vi "RT.vi"() -> ()   [LabVIEW 2025]
uses:
  Cluster.ctl
  Enum.ctl
  Conn_state.ctl
  <vilib>/FPGAPlugInAG/myRIO-1900/niLvFpga_Open_myRIO-1900.vi
  <vilib>/rvi/interface/common/dynamic/niFpgaDynamicAddResources.vi
  <vilib>/Utility/error.llb/Error Cluster From Error Code.vi
  <vilib>/rvi/errors/niLvFpgaAdjustHostInterfaceError.vi
  <vilib>/FPGAPlugInAG/Dynamic/niLvFpga_Close_Dynamic.vi
  <vilib>/rvi/interface/nirviOpenFPGA/nirviOpenFPGA.xnode
  FPGA Bitfiles/andrzejkozdrowsk_FPGATarget_fpgamain_Nau7SJ+XEAg.lvbitx
  <vilib>/rvi/interface/nirviReadWriteControl/nirviReadWriteControl.xnode
  <vilib>/rvi/interface/nirviCloseFPGA/nirviCloseFPGA.xnode
  <vilib>/rvi/interface/Simulation/niFpgaSimulationCallBeginRW.vi
  <resource>/objmgr/ni.dex.rc
  NiFpgaLv.dll
panel:
  in  "Acc_delay":u16=500
  out "Is Connected":bool
  out "Stop":bool
  out "Acc_Data":i16[](graph)
  out "error out":errorcluster
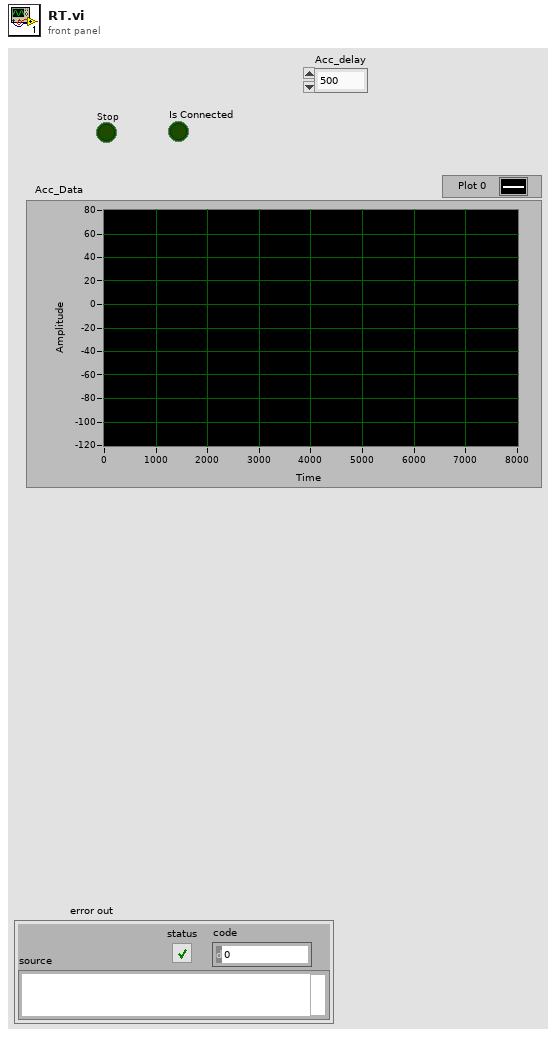
[diagram p1: front panel]
types:
  T1 = typedef "Conn_state.ctl" = enum16{"Disconected", "Reconecting", "Connected"}
  T2 = typedef "Cluster.ctl" = cluster{"X":u32, "Stop":bool, "Y":u32, "Z":u32, "Trigger":bool, "Select":T3}
  T3 = typedef "Enum.ctl" = enum16{"Trigger", "Stop", "Z", "Y", "X"}
  T4 = cluster{"Threshold_X":i16, "Threshold_Y":i16, "Threshold_Z":i16, "Trigger":bool}
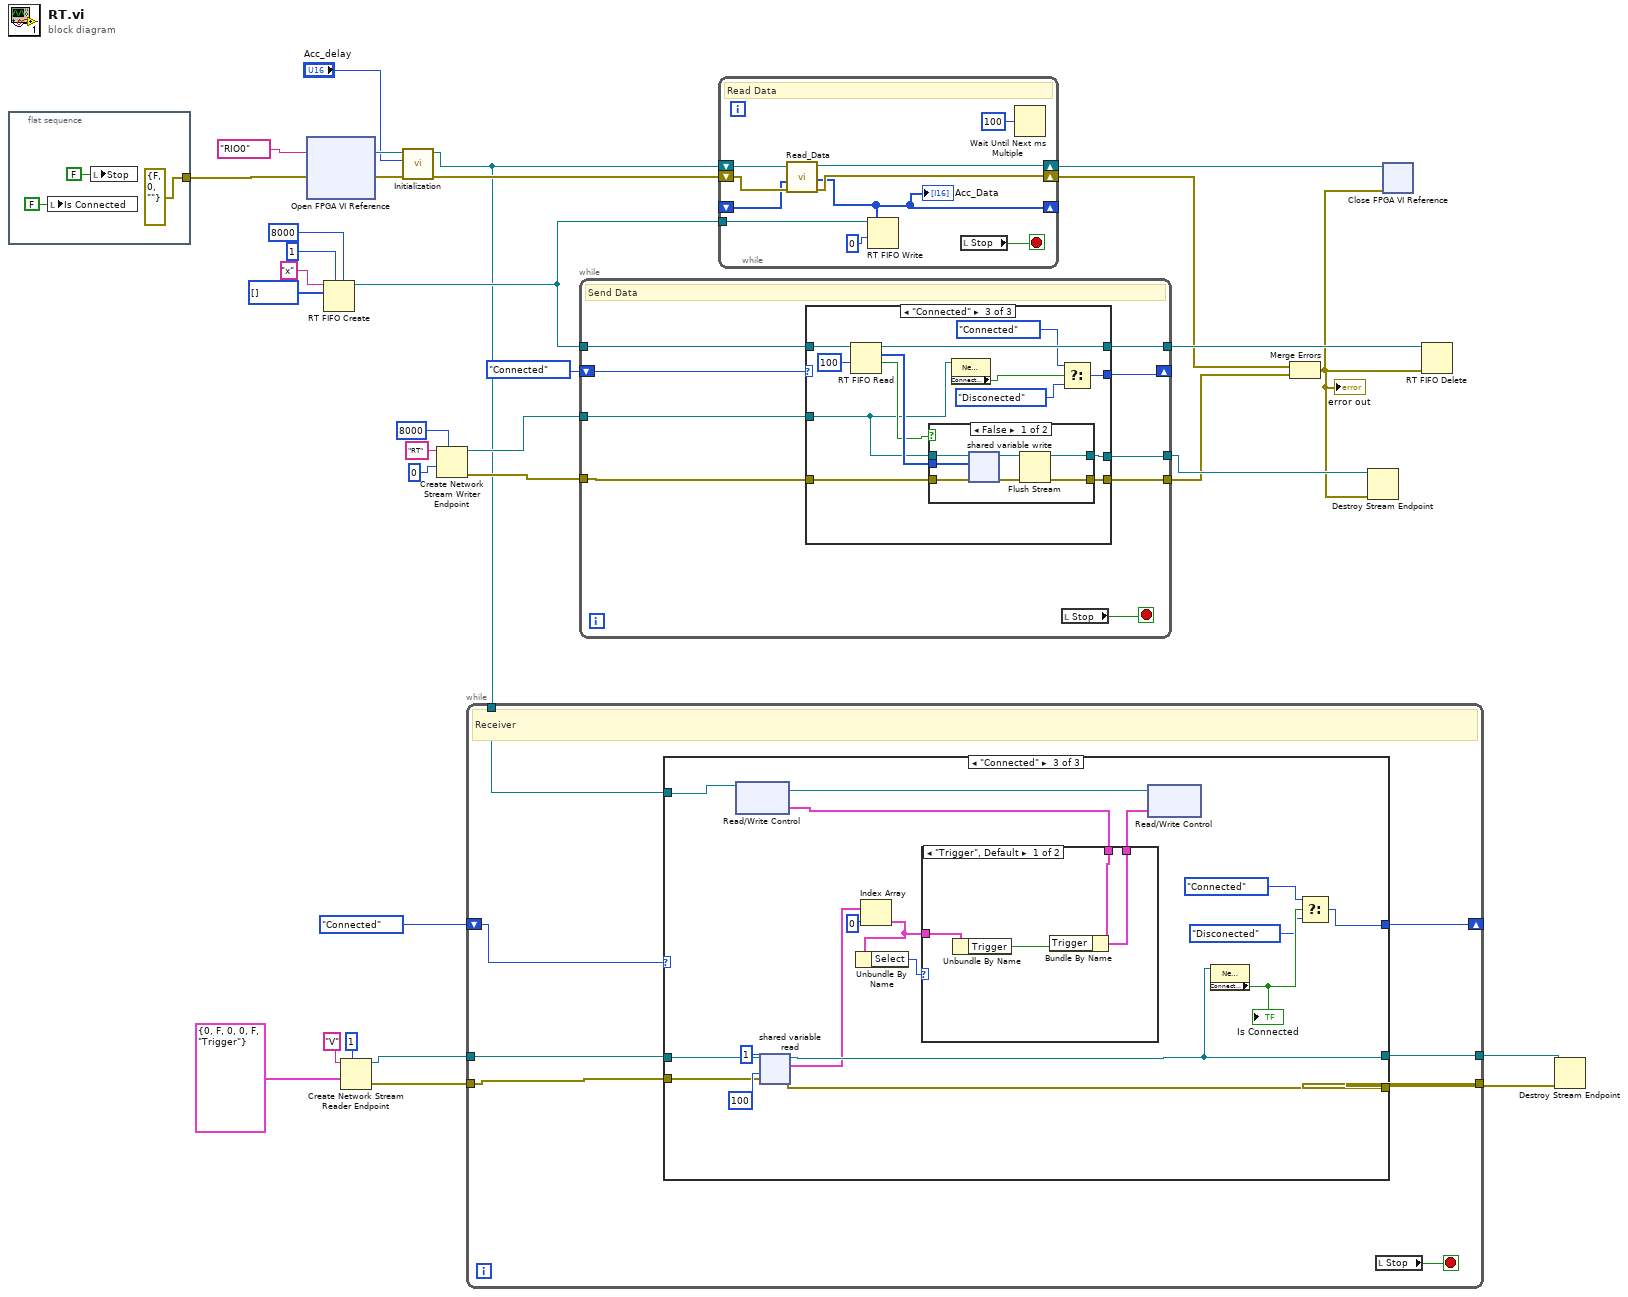
[diagram p0: block diagram]
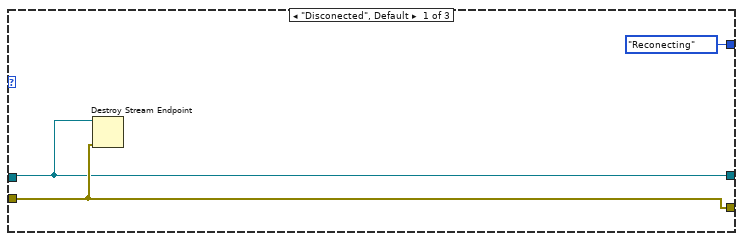
[diagram p2: hidden frame]
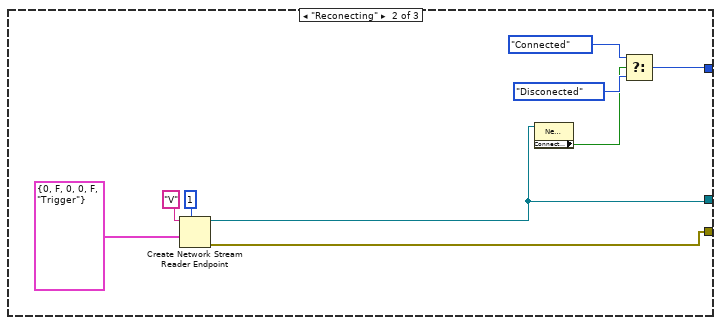
[diagram p3: hidden frame]
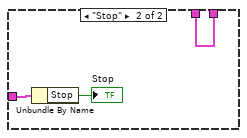
[diagram p4: hidden frame]
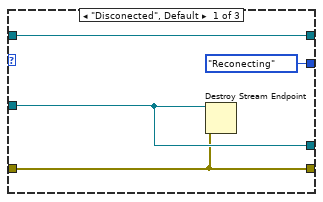
[diagram p5: hidden frame]
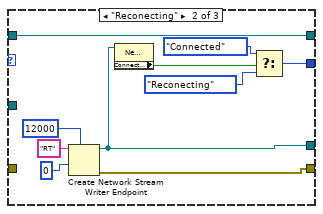
[diagram p6: hidden frame]
diagram:
  n1 = flat-sequence {
    tunnel: [errorcluster {"status"=FALSE, "code"=0, "source"=""} ("error in")] -> w21
    frame #0 {
      n2 = local write "Is Connected"(FALSE ("Is Connected")) -> ()
      n3 = local write "Stop"(FALSE ("Stop")) -> ()
    }
  }
  n4 = xnode "Open FPGA VI Reference"("error in"=w21, "resource name"=tag "RIO0") -> ("FPGA VI Reference Out"=w3:refnum<k20>, "error out"=w24:errorcluster)
  n5 = RT FIFO Create(0:"x" ("name (unnamed)"), 1:i32[] [], 4:u32 1 ("size (10)"), 6:u32 8000 ("elements in array (1)")) -> (8:w27:refnum<k33>)  [unwired: 4 in, 2 out]
  n6 = Create Network Stream Reader Endpoint(7:1 ("reader buffer size"), 9:T2 {"X"=0, "Stop"=FALSE, "Y"=0, "Z"=0, "Trigger"=FALSE, "Select"=enum."Trigger"} ("Variable"), 11:"V" ("reader name")) -> (0:w7:errorcluster, 3:w8:refnum<k21>)  [unwired: 4 in]
  n7 = call "Initialization.vi"("error in"=w24, "Acc_delay"="Acc_delay", "FPGA VI Reference In"=w3) -> ("error out"=w23:errorcluster, "FPGA VI Reference Out"=w2:refnum<k20>)  [unwired: 7 in]
  n8 = Create Network Stream Writer Endpoint(7:8000 ("writer buffer size"), 9:0, 11:"RT" ("writer name")) -> (0:w14:errorcluster, 3:w16:refnum<k21>)  [unwired: 4 in]
  n9 = while {
    tunnel: w2 -> [w43]
    tunnel: [w38] -> w12
    tunnel: [w41] -> w11
    tunnel: w7 -> [w40]
    tunnel: w8 -> [w39]
    shift-right: [w36] -> _
    shift-left: Conn_state."Connected" ("Conn_state") -> [w37]
    stop <- w42 stop-if-true
    # "Receiver"
    n10 = case shown="\"Connected\"" w37 {
      tunnel: w43 -> [_ _ w73]
      tunnel: [w44 w48 w64] -> w38
      tunnel: [w45 w47 w63] -> w41
      tunnel: w40 -> [w45 _ w62]
      tunnel: w39 -> [w44 _ w60]
      tunnel: [Conn_state."Reconecting" ("Conn_state") w52 w56] -> w36
      frame "Disconected", Default {
        n11 = Destroy Stream Endpoint(8:w45, 11:w44) -> ()  [unwired: 1 out]
      }
      frame "Reconecting" {
        n12 = Create Network Stream Reader Endpoint(7:1 ("reader buffer size"), 9:T2 {"X"=0, "Stop"=FALSE, "Y"=0, "Z"=0, "Trigger"=FALSE, "Select"=enum."Trigger"} ("Variable"), 11:"V" ("reader name")) -> (0:w47:errorcluster, 3:w48:refnum<k21>)  [unwired: 4 in]
        n13 = property class="Network Stream Endpoint"(reference=w48) -> ("Connected"=w53:bool)  [unwired: 1 in, 2 out]
        n14 = Select(t=Conn_state."Connected" ("Conn_state"), s=w53, f=Conn_state."Disconected" ("Conn_state")) -> (s? t:f=w52:T1)
      }
      frame "Connected" {
        n15 = xnode "Read/Write Control"("FPGA VI Reference In"=w73) -> ("FPGA VI Reference Out"=w70:refnum<k20>, "Data"=w69:T4)  [unwired: 1 in, 1 out]
        n16 = shared-variable-read(w60, w62, 100 ("timeout ms (-1)"), 1 ("# elements")) -> (w64:refnum<k21>, w63:errorcluster, w61:T2[])  [unwired: 1 out]
        n17 = Index Array(array=w61, index=0) -> (element=w67:T2)
        n18 = Unbundle By Name(w67) -> ("Select"=w66:T3)
        n19 = case shown="\"Trigger\", Default" w66 {
          tunnel: [w75 w78] -> w65
          tunnel: w67 -> [w77 w80]
          tunnel: w69 -> [w74 w78]
          frame "Trigger", Default {
            n20 = Unbundle By Name(w77) -> ("Trigger"=w76:bool)
            n21 = Bundle By Name(cluster=w74, "Trigger"=w76) -> (w75:T4)
          }
          frame "Stop" {
            n22 = Unbundle By Name(w80) -> ("Stop"=→"Stop":bool)
          }
        }
        n23 = xnode "Read/Write Control"("FPGA VI Reference In"=w70, "Data"=w65) -> ()  [unwired: 1 in, 2 out]
        n24 = property class="Network Stream Endpoint"(reference=w64) -> ("Connected"=w59:bool)  [unwired: 1 in, 2 out]
        "Is Connected" <- w59
        n25 = Select(t=Conn_state."Connected" ("Conn_state"), s=w59, f=Conn_state."Disconected" ("Conn_state")) -> (s? t:f=w56:T1)
      }
    }
    n26 = local read "Stop"() -> (w42:bool)
  }
  n27 = while {
    tunnel: w27 -> [w89]
    tunnel: [w88] -> w28
    shift-right: [w85] -> _
    shift-left: Conn_state."Connected" ("Conn_state") -> [w86]
    tunnel: w16 -> [w84]
    tunnel: [w83] -> w15
    tunnel: w14 -> [w82]
    tunnel: [w81] -> w13
    stop <- w87 stop-if-true
    # "Send Data"
    n28 = case shown="\"Connected\"" w86 {
      tunnel: w89 -> [w93 w102 w116]
      tunnel: w82 -> [w90 _ w115]
      tunnel: [w91 w94 w114] -> w83
      tunnel: [w93 w102 w113] -> w88
      tunnel: [w90 w95 w112] -> w81
      tunnel: w84 -> [w91 _ w108]
      tunnel: [Conn_state."Reconecting" ("Conn_state") w103 w104] -> w85
      frame "Disconected", Default {
        n29 = Destroy Stream Endpoint(8:w90, 11:w91) -> ()  [unwired: 1 out]
      }
      frame "Reconecting" {
        n30 = Create Network Stream Writer Endpoint(7:12000 ("writer buffer size"), 9:0, 11:"RT" ("writer name")) -> (0:w95:errorcluster, 3:w94:refnum<k21>)  [unwired: 4 in]
        n31 = property class="Network Stream Endpoint"(reference=w94) -> ("Connected"=w101:bool)  [unwired: 1 in, 2 out]
        n32 = Select(t=Conn_state."Connected" ("Conn_state"), s=w101, f=Conn_state."Reconecting" ("Conn_state")) -> (s? t:f=w103:T1)
      }
      frame "Connected" {
        n33 = RT FIFO Read(0:w116, 2:100 ("timeout in ms (0)")) -> (8:w113:refnum<k33>, 9:w111:i32[], 10:w109:bool)  [unwired: 2 in, 2 out]
        n34 = case shown="False" w109 {
          tunnel: w111 -> [w123 _]
          tunnel: w115 -> [w120 w124]
          tunnel: w108 -> [w119 w125]
          tunnel: [w118 w125] -> w114
          tunnel: [w117 w124] -> w112
          frame False {
            n35 = shared-variable-write(w119, w120, w123) -> (w122:refnum<k21>, w121:errorcluster)  [unwired: 1 in, 1 out]
            n36 = Flush Stream(8:w121, 11:w122) -> (0:w117:errorcluster, 3:w118:refnum<k21>)  [unwired: 2 in, 1 out]
          }
          frame True {
          }
        }
        n37 = property class="Network Stream Endpoint"(reference=w108) -> ("Connected"=w107:bool)  [unwired: 1 in, 2 out]
        n38 = Select(t=Conn_state."Connected" ("Conn_state"), s=w107, f=Conn_state."Disconected" ("Conn_state")) -> (s? t:f=w104:T1)
      }
    }
    n39 = local read "Stop"() -> (w87:bool)
  }
  n40 = while {
    shift-right: [w126] -> w26
    shift-left: w2 -> [w127]
    shift-right: [w133] -> w25
    shift-left: w23 -> [w132]
    tunnel: w27 -> [w134]
    shift-right: [w129] -> _
    shift-left: _ -> [w131]
    stop <- w128 stop-if-true
    # "Read Data"
    n41 = call "Read_Data.vi"("error in"=w132, "Shift_Register_In"=w131, "FPGA VI Reference In"=w127) -> ("error out"=w133:errorcluster, "Shift_Register_Out"=w129:i16[], "FPGA VI Reference Out 2"=w126:refnum<k20>)  [unwired: 6 in]
    "Acc_Data" <- w129
    n42 = RT FIFO Write(0:w134, 1:w129, 2:0 ("timeout in ms (0)")) -> ()  [unwired: 2 in, 4 out]
    n43 = local read "Stop"() -> (w128:bool)
    n44 = Wait Until Next ms Multiple(millisecond multiple=u32 100) -> ()  [unwired: 1 out]
  }
  n45 = Merge Errors(w25, w13) -> (w4:errorcluster)
  "error out" <- w4
  n46 = Destroy Stream Endpoint(8:w4, 11:w15) -> ()  [unwired: 1 out]
  n47 = xnode "Close FPGA VI Reference"("FPGA VI Reference In"=w26, "error in"=w4) -> ()  [unwired: 1 out]
  n48 = RT FIFO Delete(0:w28, 3:w4) -> ()  [unwired: 1 in, 1 out]
  n49 = Destroy Stream Endpoint(8:w11, 11:w12) -> ()  [unwired: 1 out]
